vi "ExFileReadNDisplay.vi"() -> ()   [LabVIEW 2010]
panel:
  in  "Full File Name":path
  in  "?":bool
  in  "FileType":u32=67371008
  out "error out":errorcluster
  in  "error in (no error)":errorcluster
  # "ExReadFileNDisplay.vi\nThis example will read in a file of the\nselected data type and display all frames.\nWhen finished viewing data, make sure to\nuse the STOP button to close the display."
  # "File Types:\nSPE = 67371008\nTIF   = 67174400\nPMI  = 67436544"
  # "Browse match pattern is set to *.spe.  Modify this if different file type is needed."
  # "This will properly close\nthe image and\ndeallocate memory."
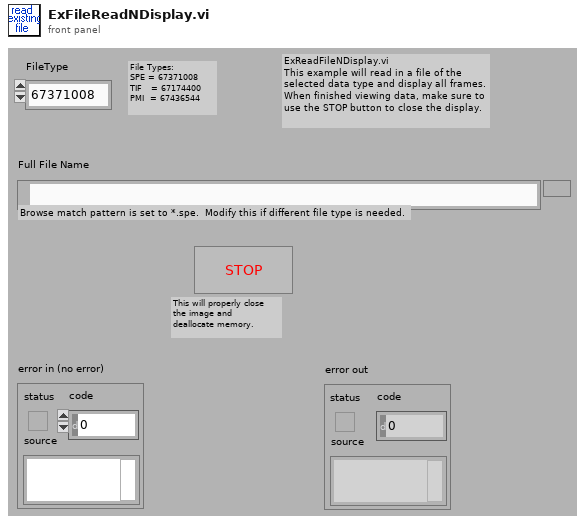
[diagram p1: front panel]
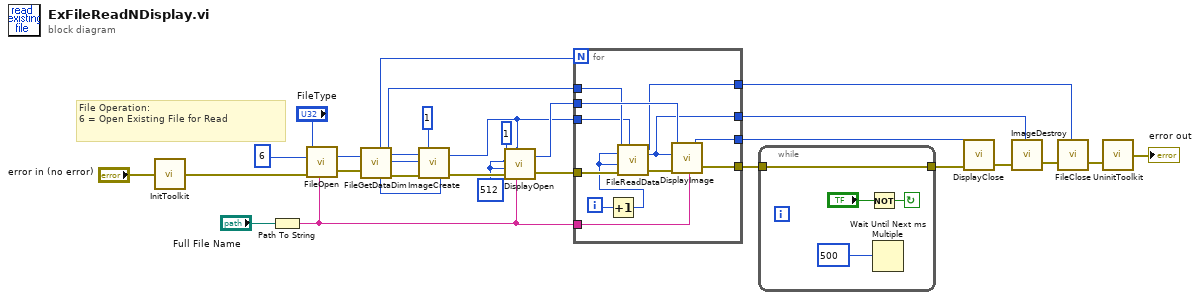
[diagram p0: block diagram]
diagram:
  w17 = 512
  # "File Operation:\n6 = Open Existing File for Read"
  n1 = call <userlib>:"InitToolkit.vi"("error in"="error in (no error)") -> ("error out"=w28:errorcluster)
  n2 = Path To String(path="Full File Name") -> (string=w1:string)
  n3 = call <userlib>:"FileOpen.vi"("error in"=w28, "File Operations"=u32 6 ("File Operation"), "FileName"=w1, "File Type"="FileType") -> ("error out"=w26:errorcluster, "File Handle"=w25:u32)
  n4 = call <userlib>:"FileGetDataDim.vi"("File Handle"=w25, "error in"=w26) -> ("Number of Frames"=w19:u32, "Data Type"=w21:u32, "File Handle"=w13:u32, "X dim"=w23:u32, "Y dim"=w22:u32, "error out"=w24:errorcluster)
  n5 = call <userlib>:"ImageCreate.vi"("X dimension"=w23, "Y dimension"=w22, "Data Type"=w21, "error in"=w24, "Number Of Frames"=1) -> ("Image Handle"=w12:u32, "error out"=w20:errorcluster)
  n6 = call <userlib>:"DisplayOpen.vi"("Display Title"=w1, "Image Handle"=w12, "error in"=w20, "Display Height"=w17, "Display Width"=w17, "Display Type"=1) -> ("error out"=w15:errorcluster, "Display Handle"=w14:u32)
  n7 = for {
    N: w19 -> [_]
    tunnel: w15 -> [w42]
    tunnel: w14 -> [w40]
    tunnel: w13 -> [w39]
    tunnel: w12 -> [w38]
    tunnel: [w35] -> w3
    tunnel: [w34] -> w11
    tunnel: [w33] -> w10
    tunnel: [w32] -> w7
    tunnel: w1 -> [w31]
    i -> [w37]
    n8 = Increment(x=w37) -> (x+1=w36:i32)
    n9 = call <userlib>:"FileReadData.vi"("File Handle"=w39, "Start Frame"=w36, "End Frame"=w36, "error in"=w42, "Image Handle"=w38) -> ("File Handle"=w33:u32, "Image Handle"=w32:u32, "error out"=w41:errorcluster)
    n10 = call <userlib>:"DisplayImage.vi"("error in"=w41, "Title"=w31, "Image Handle"=w32, "Display Handle"=w40) -> ("error out"=w35:errorcluster, "Display Handle"=w34:u32)
  }
  n11 = while {
    tunnel: w3 -> [w46]
    tunnel: [w46] -> w4
    stop <- w44 continue-if-true
    n12 = Not(x="?") -> (.not. x?=w44:bool)
    n13 = Wait Until Next ms Multiple(millisecond multiple=500) -> ()  [unwired: 1 out]
  }
  n14 = call <userlib>:"DisplayClose.vi"("error in"=w4, "Display Handle"=w11) -> ("error out"=w9:errorcluster)
  n15 = call <userlib>:"ImageDestroy.vi"("error in"=w9, "Data handle"=w7) -> ("error out"=w8:errorcluster)
  n16 = call <userlib>:"FileClose.vi"("error in"=w8, "File Handle"=w10) -> ("error out"=w6:errorcluster)
  n17 = call <userlib>:"UninitToolkit.vi"("error in"=w6) -> ("error out"=→"error out":errorcluster)
